vi "Robot Global Data.vi"() -> ()   [LabVIEW 2020]
doc: "This global VI can contain as many global variables as you need. Place a control on the panel, give it a good name. To read or write to it from a VI, drag the icon to the diagram of that VI. You can also drag from the project. Click on the node to change which global you access. You shouldn't have multiple locations writing to a global or it will cause a race-condition."
uses:
  <vilib>/Rock Robotics/WPI/Camera/WPI_CameraImageSize.ctl
  <vilib>/Rock Robotics/WPI/DriverStation/WPI_DriverStationRobotMode2.ctl
panel:
  in  "Rotate Complete":bool
  in  "Current Bar":dbl
  in  "Climb Complete":bool
  in  "Extend Complete":bool
  in  "Climb Guard":bool
  in  "Manual Clamp":bool
  in  "Manual Rotate In":bool
  in  "Manual Rotate Out":bool
  in  "Manual Retract":bool
  in  "Manual Extend":bool
  in  "Manual Right":bool
  in  "Manual Left":bool
  in  "Climb Transversal":bool
  in  "Climb High":bool
  in  "Climb Mid":bool
  in  "Climb Low":bool
  in  "Abort":bool
  in  "Proceed":bool
  in  "Backward To Stripe":bool
  in  "Forward To Stripe":bool
  in  "auto aim":bool
  in  "Shoot":bool
  in  "Intake":bool
  in  "Robot Mode":T1
  in  "image size":T2=enum."320x240"
  in  "Enable Vision":bool
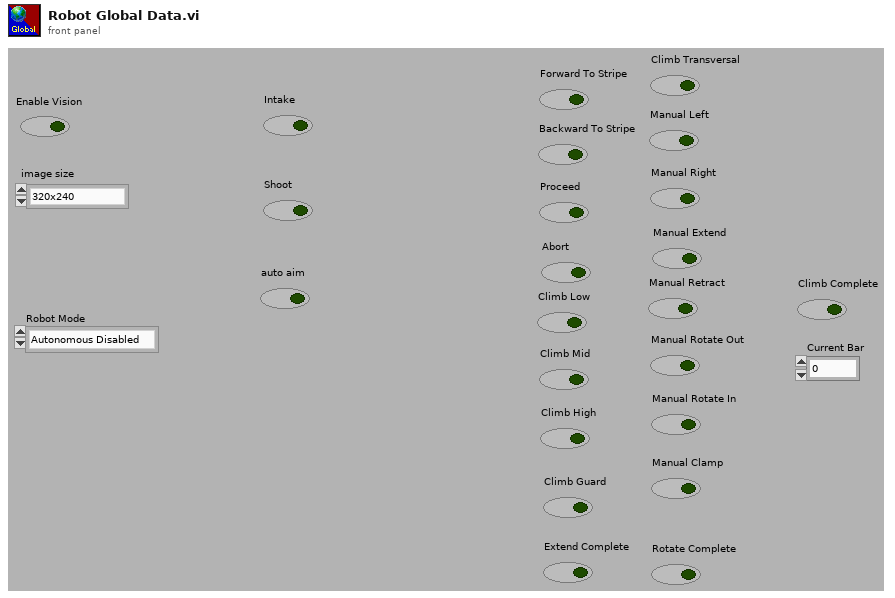
[diagram p1: front panel]
types:
  T1 = typedef "WPI_DriverStationRobotMode2.ctl" = enum16{"Autonomous Disabled", "Autonomous Enabled", "Teleop Disabled", "Teleop Enabled", "Disconnected", "Finish", "Test Disabled", "Test Enabled", "Emergency Stopped"}
  T2 = typedef "WPI_CameraImageSize.ctl" = enum16{"640x480", "320x240", "160x120", "Custom"}
diagram:
